vi "initialize.vi"(0 "HGF_SVCommand in":refnum<class "HGF_SVCommand.lvclass">, 3 "initializationData":variant, 5 "error in (no error)":errorcluster, 7 "binaryString":string, 8 "I8 Array":i8[](array[numeric]), 9 "prependSize? (T)":bool, 11 "byteOrder (0:big-endian, network order)":T1(ring)) -> (14 "HGF_SVCommand out":refnum<class "HGF_SVCommand.lvclass">, 17 "found?":bool, 19 "error out":errorcluster)   [LabVIEW 2012, in "HGF_SV.lvlib" / "HGF_SVCommand.lvclass"]
uses:
  HGF_SVCommand.lvclass
  HGF_BaseClasses/HGF_PVSubscriber/HGF_PVSubscriber.lvclass
  HGF_SVCommand.lvclass/HGF_SVCommand.ctl
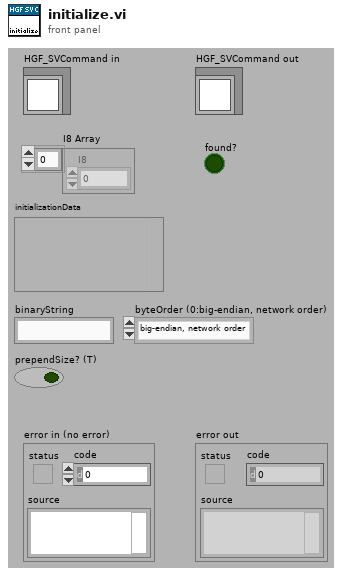
[diagram p1: front panel]
types:
  T1 = enum16{"big-endian, network order", "native, host order", "little-endian"}
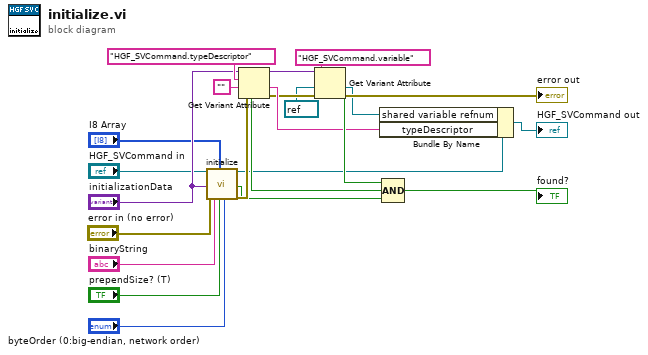
[diagram p0: block diagram]
diagram:
  n1 = call-parent "initialize.vi"("HGV_PVBase"="HGF_SVCommand in", "initializationData"="initializationData", "error in (no error)"="error in (no error)", "binaryString"="binaryString", "I8 Array"="I8 Array", "prependSize? (T)"="prependSize? (T)", "byteOrder (0:big-endian, network order)"="byteOrder (0:big-endian, network order)") -> ("HGV_PVBase"=w8:refnum<class "HGF_SVCommand.lvclass">, "found?"=w19:bool, "error out"=w21:errorcluster)  [unwired: 10 out]
  n2 = Get Variant Attribute(Variant="initializationData", name="HGF_SVCommand.typeDescriptor", default value (empty Variant)="", error in=w21) -> (duplicate Variant=w4:variant, found=w18:bool, value=w5:string, error out=w3:errorcluster)
  n3 = Get Variant Attribute(Variant=w4, name="HGF_SVCommand.variable", default value (empty Variant)=refnum<k21> refnum ("shared variable refnum"), error in=w3) -> (found=w22:bool, value=w1:refnum<k21>, error out=→"error out":errorcluster)  [unwired: 1 out]
  n4 = Bundle By Name(cluster=w8, "shared variable refnum"=w1, "typeDescriptor"=w5) -> (→"HGF_SVCommand out":refnum<class "HGF_SVCommand.lvclass">)
  n5 = Compound Arithmetic op=AND(w22, w18, w19) -> (→"found?":bool)
